vi "Meas Generate Sequence.vi"(7 "processing setup":T1, 8 "error in":errorcluster, 11 "sequence setup":T7) -> (0 "error out":errorcluster, 2 "sequence size":i32, 3 "sequence out":T15[](array[typedef]))   [LabVIEW 2013]
doc: "Builds measurement sequence. It will take vector of measurement configurations (groups) and for each group it will generate 'average cycles' measurements with the same configuration. All measurements are merged into a single sequence. Sequence will also contain control flags for sequencer ('adc modified?', 'group done?', etc.). The VI also generates file names/paths for the data files and header files."
uses:
  Meas Sequence Item.ctl
  Meas Sampling Configuration.ctl
  adc/ADC Trig Config.ctl
  adc/ADC Trig Mode Source.ctl
  adc/ADC Trig Coupling.ctl
  adc/ADC Trig Slope.ctl
  processing/QWTB/Meas Proc QWTB Algorithm Parameter Data.ctl
  Meas Sequence Configuration.ctl
  Meas Range Mode.ctl
  Meas Sampling Rate Mode.ctl
  processing/Meas Process Config.ctl
  processing/Meas Process Mode.ctl
  processing/Meas Process Raw Config.ctl
  processing/Meas Process Raw Result Mode.ctl
  processing/QWTB/Meas Proc QWTB Setup.ctl
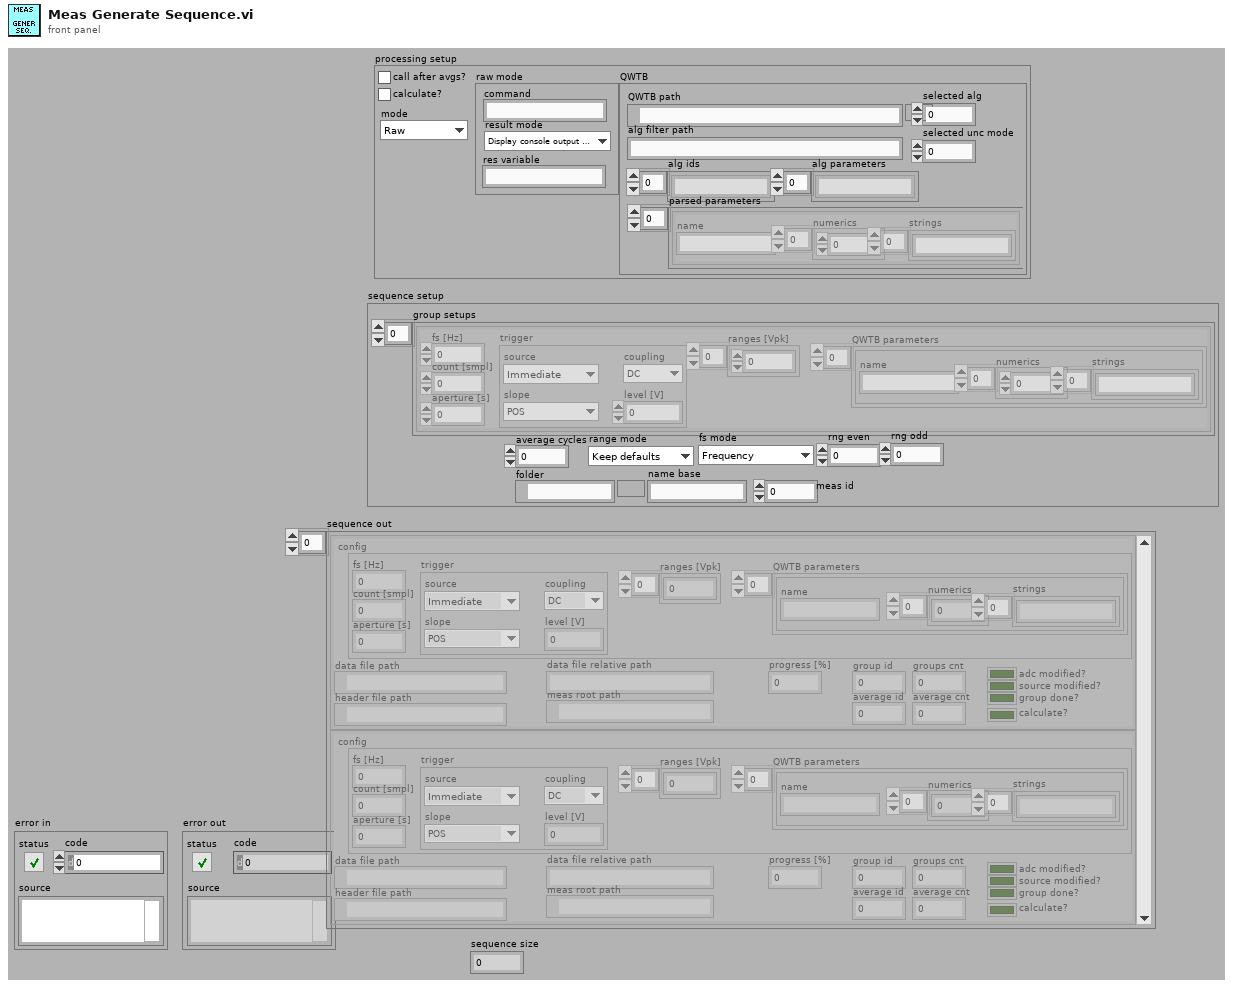
[diagram p1: front panel]
types:
  T1 = typedef "Meas Process Config.ctl" = cluster{"mode":T2, "call after avgs?":bool, "calculate?":bool, "raw mode":T3, "QWTB":T5}
  T2 = typedef "Meas Process Mode.ctl" = enum16{"Raw", "QWTB"}
  T3 = typedef "Meas Process Raw Config.ctl" = cluster{"command":string, "result mode":T4, "res variable":string}
  T4 = typedef "Meas Process Raw Result Mode.ctl" = enum16{"Display console output (only Octave)", "Display string variable", "Display result file %respath%"}
  T5 = typedef "Meas Proc QWTB Setup.ctl" = cluster{"QWTB path":path, "alg filter path":string, "alg ids":string[], "alg parameters":string[], "parsed parameters":T6[], "selected alg":i32, "selected unc mode":i32}
  T6 = typedef "Meas Proc QWTB Algorithm Parameter Data.ctl" = cluster{"name":string, "numerics":dbl[], "strings":string[]}
  T7 = typedef "Meas Sequence Configuration.ctl" = cluster{"group setups":T8[], "average cycles":i32, "range mode":T13, "fs mode":T14, "rng even":dbl, "rng odd":dbl, "folder":path, "name base":string, "meas id":i32}
  T8 = typedef "Meas Sampling Configuration.ctl" = cluster{"fs [Hz]":dbl, "count [smpl]":i64, "aperture [s]":dbl, "trigger":T9, "ranges [Vpk]":dbl[], "QWTB parameters":T6[]}
  T9 = typedef "ADC Trig Config.ctl" = cluster{"source":T10, "level [V]":dbl, "coupling":T11, "slope":T12}
  T10 = typedef "ADC Trig Mode Source.ctl" = enum16{"Immediate", "External", "Level"}
  T11 = typedef "ADC Trig Coupling.ctl" = enum16{"DC", "AC"}
  T12 = typedef "ADC Trig Slope.ctl" = enum16{"POS", "NEG"}
  T13 = typedef "Meas Range Mode.ctl" = enum16{"Keep defaults", "Set All channels", "Set Odd and Even channels"}
  T14 = typedef "Meas Sampling Rate Mode.ctl" = enum16{"Frequency", "Period"}
  T15 = typedef "Meas Sequence Item.ctl" = cluster{"config":T8, "data file path":path, "header file path":path, "group id":i32, "average id":i32, "group done?":bool, "adc modified?":bool, "source modified?":bool, "progress [%]":dbl, "groups cnt":i32, "average cnt":i32, "data file relative path":string, "meas root path":path, "calculate?":bool}
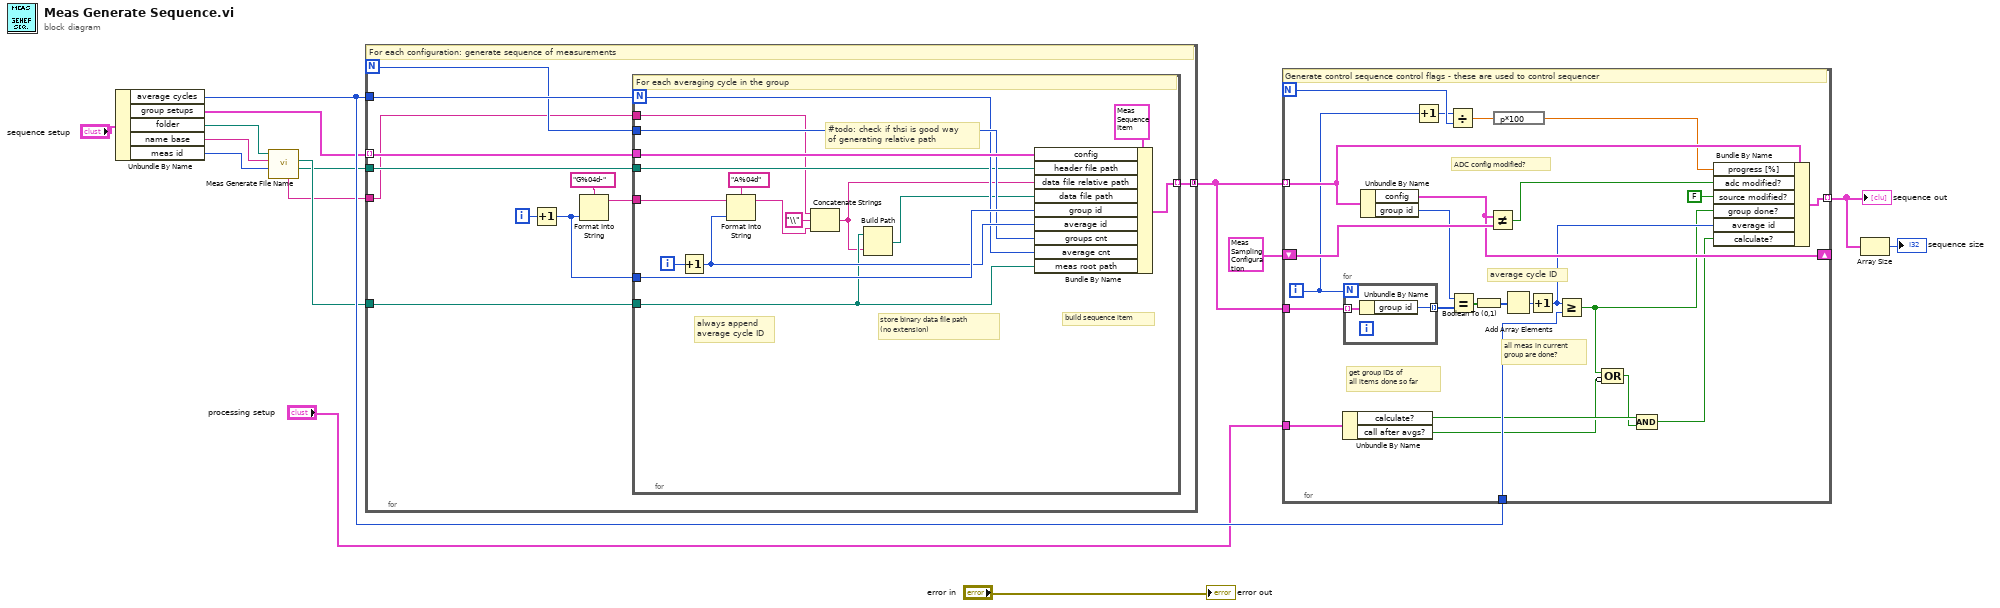
[diagram p0: block diagram]
diagram:
  n1 = Unbundle By Name("sequence setup") -> ("average cycles"=w9:i32, "group setups"=w8:T8[], "folder"=w7:path, "name base"=w6:string, "meas id"=w5:i32)
  n2 = call "Meas Generate File Name.vi"("meas id"=w5, "name base"=w6, "folder"=w7) -> ("header file full path"=w3:path, "measurement root folder"=w4:path, "waveforms folder out"=w2:string)  [unwired: 4 in, 2 out]
  n3 = for {
    N -> [w19]
    tunnel: w8 -> [w18] mode=indexing
    tunnel: w4 -> [w21]
    tunnel: [w24] -> w14 mode=concatenating
    tunnel: w9 -> [w23]
    tunnel: w3 -> [w20]
    tunnel: w2 -> [w17]
    i -> [w25]
    # "For each configuration: generate sequence of measurements"
    n4 = Increment(x=w25) -> (x+1=w22:i32)
    n5 = Format Into String(format string="G%04d-", w22) -> (resulting string=w16:string)  [unwired: 2 in, 1 out]
    n6 = for {
      N: w23 -> [w35]
      tunnel: w18 -> [w42]
      tunnel: w20 -> [w34]
      tunnel: w21 -> [w32]
      tunnel: w22 -> [w39]
      tunnel: [w38] -> w24 mode=indexing
      tunnel: w19 -> [w36]
      tunnel: w16 -> [w31]
      tunnel: w17 -> [w29]
      i -> [w41]
      # "#todo: check if thsi is good way \nof generating relative path"
      # "always append\naverage cycle ID"
      # "store binary data file path\n(no extension)"
      # "build sequence item"
      # "For each averaging cycle in the group"
      n7 = Increment(x=w41) -> (x+1=w37:i32)
      n8 = Format Into String(format string="A%04d", initial string=w31, w37) -> (resulting string=w27:string)  [unwired: 1 in, 1 out]
      n9 = Concatenate Strings(w29, "\\" ("string"), w27) -> (w28:string)
      n10 = Build Path(base path=w32, name or relative path=w28) -> (appended path=w33:path)
      n11 = Bundle By Name(cluster=T15 {"config"={"fs [Hz]"=0.0, "count [smpl]"=0, "aperture [s]"=0.0, "trigger"={"source"=enum."Immediate", "level [V]"=0.0, "coupling"=enum."DC", "slope"=enum."POS"}, "ranges [Vpk]"=[], "QWTB parameters"=[]}, "data file path"=path "", "header file path"=path "", "group id"=0, "average id"=0, "group done?"=FALSE, "adc modified?"=FALSE, "source modified?"=FALSE, "progress [%]"=0.0, "groups cnt"=0, "average cnt"=0, "data file relative path"="", "meas root path"=path "", "calculate?"=FALSE} ("sequence item"), "config"=w42, "header file path"=w34, "data file relative path"=w28, "data file path"=w33, "group id"=w39, "average id"=w37, "groups cnt"=w36, "average cnt"=w35, "meas root path"=w32) -> (w38:T15)
    }
  }
  n12 = for {
    N -> [w51]
    tunnel: w14 -> [w67] mode=indexing
    shift-right: [w65] -> _
    shift-left: T8 {"fs [Hz]"=0.0, "count [smpl]"=0, "aperture [s]"=0.0, "trigger"={"source"=enum."Immediate", "level [V]"=0.0, "coupling"=enum."DC", "slope"=enum."POS"}, "ranges [Vpk]"=[], "QWTB parameters"=[]} ("config") -> [w68]
    tunnel: w14 -> [w63]
    tunnel: w9 -> [w57]
    tunnel: [w53] -> w12 mode=indexing
    tunnel: "processing setup" -> [w49]
    i -> [w55]
    # "ADC config modified?"
    # "average cycle ID"
    # "all meas in current\ngroup are done?"
    # "get group IDs of\nall items done so far"
    # "Generate control sequence control flags - these are used to control sequencer"
    n13 = Unbundle By Name(w49) -> ("calculate?"=w48:bool, "call after avgs?"=w47:bool)
    n14 = for {
      N: w55 -> [_]
      tunnel: w63 -> [w70] mode=indexing
      tunnel: [w69] -> w62 mode=indexing
      n15 = Unbundle By Name(w70) -> ("group id"=w69:i32)
    }
    n16 = Unbundle By Name(w67) -> ("config"=w65:T8, "group id"=w61:i32)
    n17 = Increment(x=w55) -> (x+1=w50:i32)
    n18 = Divide(x=w50, y=w51) -> (x/y=w54:dbl)
    n19 = Equal?(x=w61, y=w62) -> (x = y?=w60:bool[])
    n20 = Boolean To (0,1)(Boolean=w60) -> (0, 1=w59:i16[])
    n21 = Not Equal?(x=w65, y=w68) -> (x != y?=w66:bool)
    n22 = expression code="p*100"(w54) -> (w52:dbl)
    n23 = Add Array Elements(numeric array=w59) -> (sum=w58:i16)
    n24 = Increment(x=w58) -> (x+1=w56:i16)
    n25 = Greater Or Equal?(x=w56, y=w57) -> (x >= y?=w46:bool)
    n26 = Compound Arithmetic op=OR(w46, invert w47) -> (w45:bool)
    n27 = Compound Arithmetic op=AND(w48, w45) -> (w44:bool)
    n28 = Bundle By Name(cluster=w67, "progress [%]"=w52, "adc modified?"=w66, "source modified?"=FALSE, "group done?"=w46, "average id"=w56, "calculate?"=w44) -> (w53:T15)
  }
  "sequence out" <- w12
  n29 = Array Size(array=w12) -> (size(s)=→"sequence size":i32)
  "error out" <- "error in"
